vi "Create Correct Arrays.vi"(8 "Data":dbl[](array[numeric]), 9 "YCoordinates":dbl[](array[numeric]), 10 "XCoordinates":dbl[](array[numeric]), 11 "UseActuatorArray":bool[](array[boolean])) -> (0 "NewData":dbl[](array[numeric]), 1 "NewYCoordinates":dbl[](array[numeric]), 2 "NewXCoordinates":dbl[](array[numeric]))   [LabVIEW 2016, in "M1M3SupportEUI_Views.lvlib"]
uses:
  M1M3SupportEUI_Views.lvlib
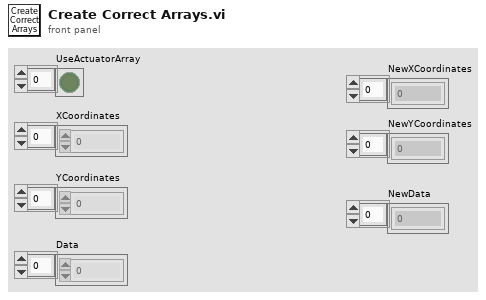
[diagram p1: front panel]
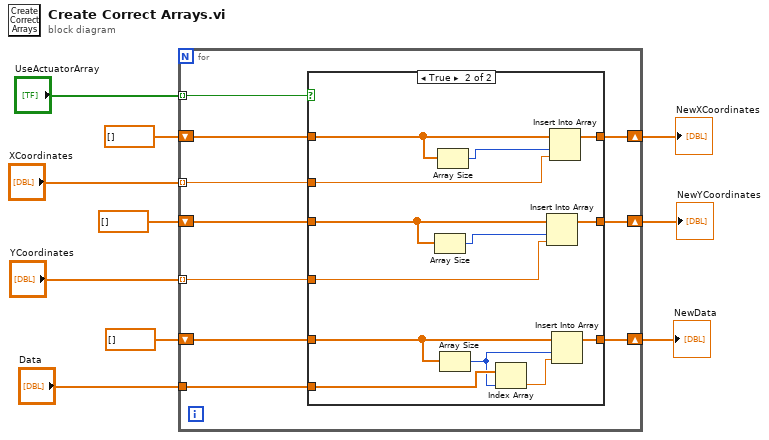
[diagram p0: block diagram]
diagram:
  n1 = for {
    tunnel: "UseActuatorArray" -> [w20] mode=indexing
    tunnel: "XCoordinates" -> [w19] mode=indexing
    tunnel: "YCoordinates" -> [w18] mode=indexing
    tunnel: "Data" -> [w11]
    shift-right: [w15] -> w1
    shift-left: dbl[] [] -> [w17]
    shift-right: [w14] -> w2
    shift-left: dbl[] [] -> [w16]
    shift-right: [w13] -> w3
    shift-left: dbl[] [] -> [w12]
    n2 = case shown="True" w20 {
      tunnel: w19 -> [_ w35]
      tunnel: w18 -> [_ w29]
      tunnel: w11 -> [_ w26]
      tunnel: w17 -> [w23 w33]
      tunnel: w16 -> [w22 w30]
      tunnel: w12 -> [w21 w27]
      tunnel: [w23 w36] -> w15
      tunnel: [w22 w31] -> w14
      tunnel: [w21 w28] -> w13
      frame False {
      }
      frame True {
        n3 = Array Size(array=w30) -> (size(s)=w32:i32)
        n4 = Array Size(array=w33) -> (size(s)=w34:i32)
        n5 = Array Size(array=w27) -> (size(s)=w25:i32)
        n6 = Index Array(array=w26, index=w25) -> (element=w24:dbl)
        n7 = Insert Into Array(array=w30, index=w32, new element=w29) -> (w31:dbl[])
        n8 = Insert Into Array(array=w33, index=w34, new element=w35) -> (w36:dbl[])
        n9 = Insert Into Array(array=w27, index=w25, new element=w24) -> (w28:dbl[])
      }
    }
  }
  "NewXCoordinates" <- w1
  "NewYCoordinates" <- w2
  "NewData" <- w3
